vi "Rectangel StraightenLineBetweenRectangles.vi"(1 "Rect1ConnectionOffset":cluster{"x":i32, "y":i32}, 2 "Rect1":T3 {"height" format="%.2f"; "width" format="%.2f"; "y" format="%.2f"; "x" format="%.2f"}, 3 "Rect2ConnectionOffset":cluster{"x":i32, "y":i32}, 4 "Rect2":T3 {"height" format="%.2f"; "width" format="%.2f"; "y" format="%.2f"; "x" format="%.2f"}, 5 "error in (no error)":errorcluster, 6 "Rect1LineDirection":T2, 7 "Rect2LineDirection":T2, 9 "path":T1[](array[typedef]) {"y" format="%.2f"; "x" format="%.2f"}) -> (14 "AdjustmentOK":bool, 15 "Rect1ConnectionOffset":cluster{"x":i32, "y":i32}, 16 "Rect2ConnectionOffset":cluster{"x":i32, "y":i32}, 19 "error out":errorcluster)   [LabVIEW 2014]
doc: "contains"
uses:
  <resource>/Framework/Providers/Open_GDS/UML/General/Rectangle/Rectangle Rectangle2D.ctl
  <resource>/Framework/Providers/Open_GDS/UML/Direction_class/DirectionTypes.ctl
  <resource>/Framework/Providers/Open_GDS/UML/General/Point/Point Point2D.ctl
  <resource>/Framework/Providers/Open_GDS/UML/Direction_class/Direction.lvclass
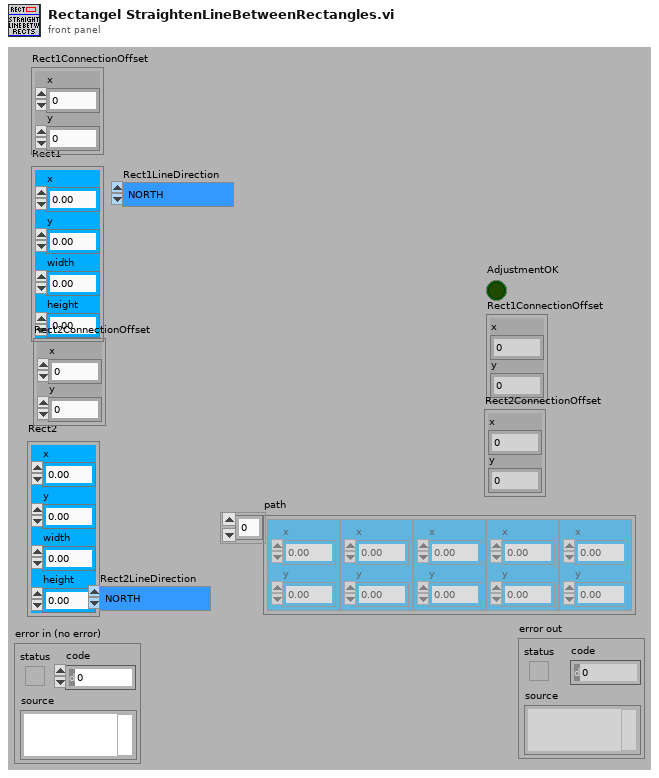
[diagram p1: front panel]
types:
  T1 = typedef "Point Point2D.ctl" = cluster{"x":dbl, "y":dbl}
  T2 = typedef "Direction.lvclass/DirectionTypes.ctl" = enum16{"NORTH", "SOUTH", "EAST", "WEST"}
  T3 = typedef "Rectangle Rectangle2D.ctl" = cluster{"x":dbl, "y":dbl, "width":dbl, "height":dbl}
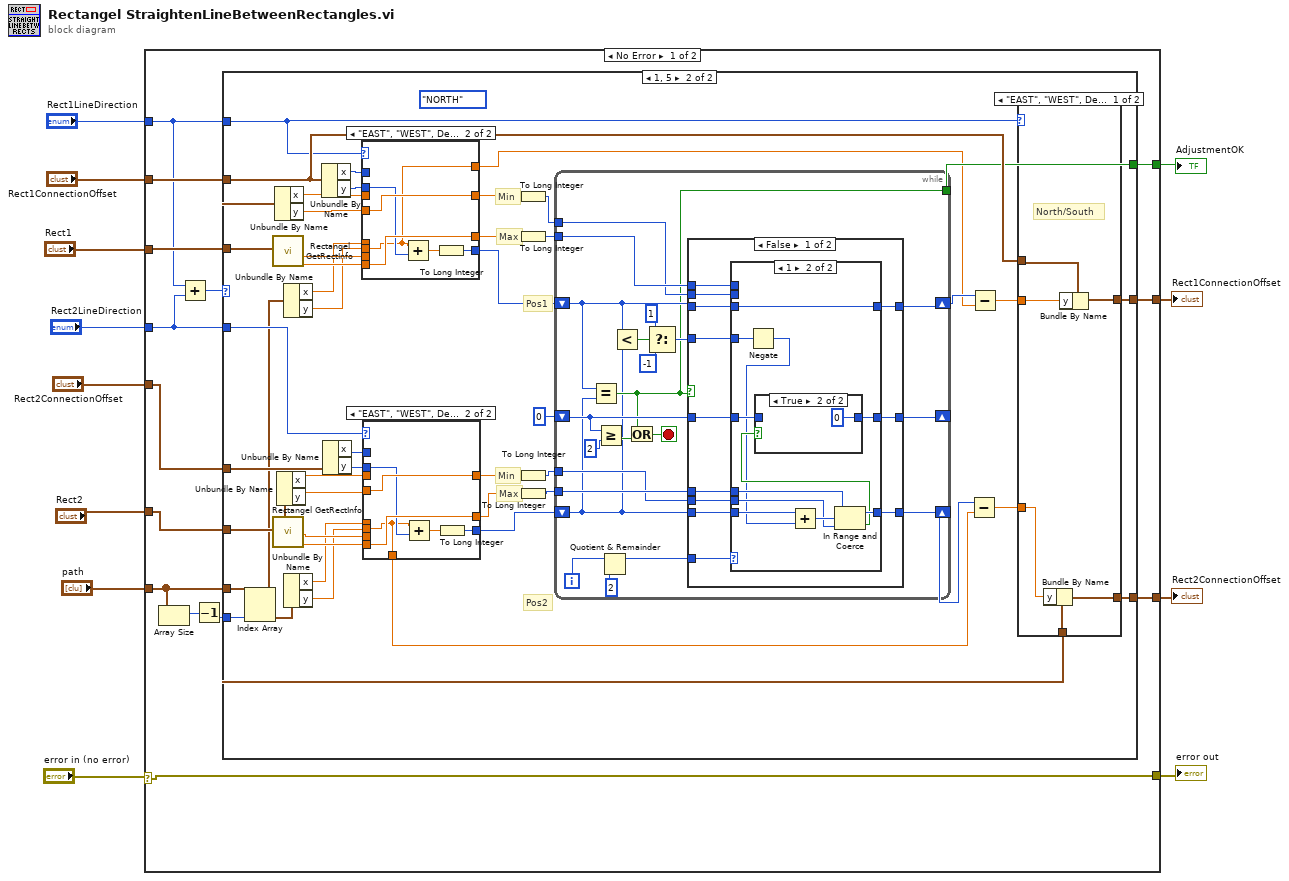
[diagram p0: block diagram]
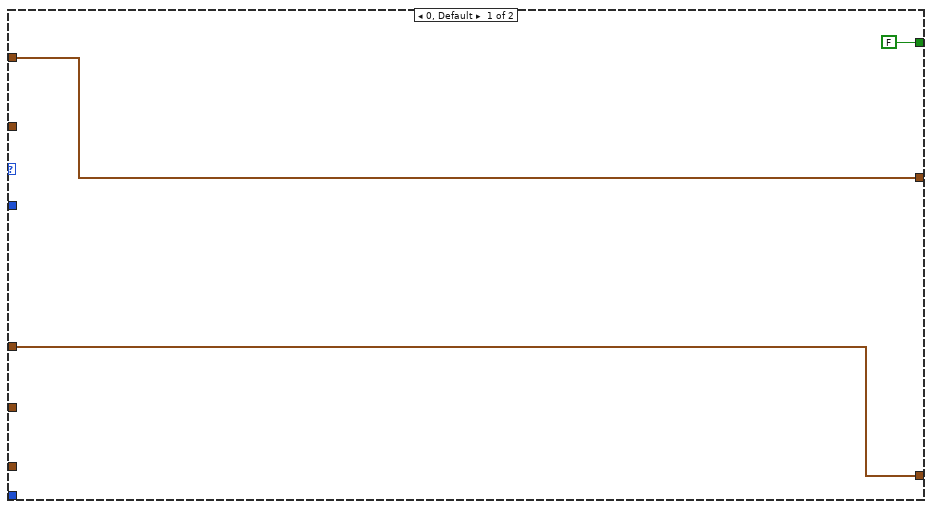
[diagram p2: hidden frame]
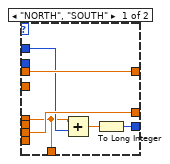
[diagram p3: hidden frame]
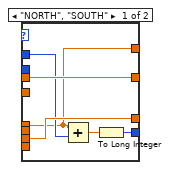
[diagram p4: hidden frame]
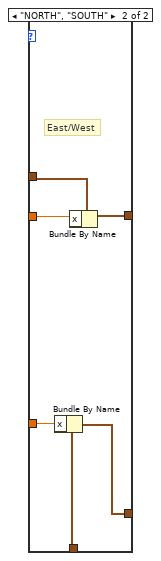
[diagram p5: hidden frame]
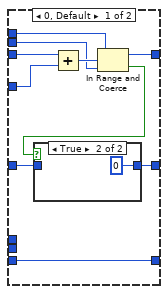
[diagram p6: hidden frame]
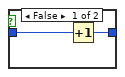
[diagram p7: hidden frame]
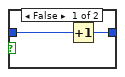
[diagram p8: hidden frame]
diagram:
  n1 = case shown="No Error" "error in (no error)" {
    selector: "error in (no error)" -> [w26 w175]
    tunnel: [w26 w175] -> w12
    tunnel: "Rect1" -> [w22 _]
    tunnel: "Rect1ConnectionOffset" -> [w23 _]
    tunnel: [w25 _] -> w8
    tunnel: "Rect2ConnectionOffset" -> [w19 _]
    tunnel: [w24 _] -> w6
    tunnel: "Rect1LineDirection" -> [w18 _]
    tunnel: [w21 _] -> w4
    tunnel: "Rect2" -> [w20 _]
    tunnel: "Rect2LineDirection" -> [w17 _]
    tunnel: "path" -> [w15 _]
    frame No Error {
      n2 = Array Size(array=w15) -> (size(s)=w14:i32)
      n3 = Add(x=w18, y=w17) -> (x+y=w16:u16)
      n4 = Decrement(x=w14) -> (x-1=w13:i32)
      n5 = case shown="1, 5" w16 {
        tunnel: [w28 w75] -> w25
        tunnel: [w27 w73] -> w24
        tunnel: w23 -> [w28 w72]
        tunnel: w22 -> [_ w70]
        tunnel: [FALSE w64] -> w21
        tunnel: w20 -> [_ w62]
        tunnel: w19 -> [w27 w61]
        tunnel: w18 -> [_ w44]
        tunnel: w17 -> [_ w51]
        tunnel: w15 -> [_ w37]
        tunnel: w13 -> [_ w36]
        frame 0, Default {
        }
        frame 1, 5 {
          (unwired) DirectionTypes."NORTH" ("Rect1LineDirection")
          # "Max"
          # "Min"
          # "Max"
          # "Min"
          # "Pos2"
          # "Pos1"
          n6 = Index Array(array=w37, index #2=w36) -> (element #1=w35:T1, element #2=w32:T1)  [unwired: 1 in]
          n7 = call <resource>:"Rectangel GetRectInfo.vi"("bounds"=w70) -> ("maxX"=w68:dbl, "maxY"=w58:dbl)  [unwired: 1 in, 16 out]
          n8 = call <resource>:"Rectangel GetRectInfo.vi"("bounds"=w62) -> ("maxX"=w53:dbl, "maxY"=w52:dbl)  [unwired: 1 in, 16 out]
          n9 = Unbundle By Name(w70) -> ("x"=w69:dbl, "y"=w59:dbl)
          n10 = Unbundle By Name(w62) -> ("x"=w55:dbl, "y"=w54:dbl)
          n11 = Unbundle By Name(w35) -> ("x"=w33:dbl, "y"=w34:dbl)
          n12 = Unbundle By Name(w32) -> ("x"=w31:dbl, "y"=w30:dbl)
          n13 = Unbundle By Name(w72) -> ("x"=w71:i32, "y"=w60:i32)
          n14 = Unbundle By Name(w61) -> ("x"=w57:i32, "y"=w56:i32)
          n15 = case shown="\"EAST\", \"WEST\", Default" w44 {
            tunnel: w71 -> [w89 _]
            tunnel: w33 -> [w88 _]
            tunnel: [w92 w98] -> w39
            tunnel: w69 -> [w91 _]
            tunnel: w68 -> [w90 _]
            tunnel: [w91 w97] -> w67
            tunnel: [w90 w96] -> w66
            tunnel: w60 -> [_ w95]
            tunnel: w59 -> [_ w97]
            tunnel: w34 -> [_ w94]
            tunnel: w58 -> [_ w96]
            tunnel: [w88 w94] -> w40
            frame "NORTH", "SOUTH" {
              n16 = Add(x=w88, y=w89) -> (x+y=w93:dbl)
              n17 = To Long Integer(number=w93) -> (32bit integer=w92:i32)
            }
            frame "EAST", "WEST", Default {
              n18 = Add(x=w94, y=w95) -> (x+y=w99:dbl)
              n19 = To Long Integer(number=w99) -> (32bit integer=w98:i32)
            }
          }
          n20 = case shown="\"EAST\", \"WEST\", Default" w51 {
            tunnel: w57 -> [w77 _]
            tunnel: w31 -> [w76 _]
            tunnel: [w80 w86] -> w41
            tunnel: w55 -> [w79 _]
            tunnel: w53 -> [w78 _]
            tunnel: [w79 w85] -> w49
            tunnel: [w78 w84] -> w48
            tunnel: w56 -> [_ w83]
            tunnel: w54 -> [_ w85]
            tunnel: w30 -> [_ w82]
            tunnel: w52 -> [_ w84]
            tunnel: [w76 w82] -> w38
            frame "NORTH", "SOUTH" {
              n21 = Add(x=w76, y=w77) -> (x+y=w81:dbl)
              n22 = To Long Integer(number=w81) -> (32bit integer=w80:i32)
            }
            frame "EAST", "WEST", Default {
              n23 = Add(x=w82, y=w83) -> (x+y=w87:dbl)
              n24 = To Long Integer(number=w87) -> (32bit integer=w86:i32)
            }
          }
          n25 = To Long Integer(number=w67) -> (32bit integer=w50:i32)
          n26 = To Long Integer(number=w66) -> (32bit integer=w65:i32)
          n27 = To Long Integer(number=w49) -> (32bit integer=w46:i32)
          n28 = To Long Integer(number=w48) -> (32bit integer=w47:i32)
          n29 = while {
            shift-right: [w122] -> w43
            shift-left: w39 -> [w129]
            shift-right: [w121] -> w42
            shift-left: w41 -> [w112]
            tunnel: w50 -> [w123]
            tunnel: w65 -> [w124]
            shift-right: [w120] -> _
            shift-left: 0 -> [w119]
            tunnel: [w115] -> w64
            tunnel: w47 -> [w114]
            tunnel: w46 -> [w113]
            i -> [w132]
            stop <- w116 stop-if-true
            n30 = Equal?(x=w129, y=w112) -> (x = y?=w115:bool)
            n31 = Greater Or Equal?(x=w119, y=2) -> (x >= y?=w117:bool)
            n32 = Quotient & Remainder(x=w132, y=2) -> (x-y*floor(x/y)=w130:i32)  [unwired: 1 out]
            n33 = Less?(x=w129, y=w112) -> (x < y?=w128:bool)
            n34 = Or(x=w115, y=w117) -> (x .or. y?=w116:bool)
            n35 = Select(t=1, s=w128, f=-1) -> (s? t:f=w125:i32)
            n36 = case shown="False" w115 {
              tunnel: w130 -> [w144 _]
              tunnel: w129 -> [w143 w172]
              tunnel: w125 -> [w142 _]
              tunnel: w124 -> [w141 _]
              tunnel: w123 -> [w140 _]
              tunnel: [w139 w172] -> w122
              tunnel: [w138 w174] -> w121
              tunnel: [w137 w173] -> w120
              tunnel: w119 -> [w136 w173]
              tunnel: w114 -> [w135 _]
              tunnel: w113 -> [w134 _]
              tunnel: w112 -> [w133 w174]
              frame False {
                n37 = case shown="1" w144 {
                  tunnel: w143 -> [w154 w158]
                  tunnel: w142 -> [w153 w160]
                  tunnel: w141 -> [w151 _]
                  tunnel: w140 -> [w150 _]
                  tunnel: [w149 w158] -> w139
                  tunnel: [w148 w167] -> w138
                  tunnel: [w145 w165] -> w137
                  tunnel: w136 -> [w146 w164]
                  tunnel: w135 -> [_ w163]
                  tunnel: w134 -> [_ w162]
                  tunnel: w133 -> [w148 w161]
                  frame 0, Default {
                    n38 = Add(x=w154, y=w153) -> (x+y=w152:i32)
                    n39 = In Range and Coerce(upper limit=w151, x=w152, lower limit=w150) -> (coerced(x)=w149:i32, In Range?=w147:bool)
                    n40 = case shown="True" w147 {
                      tunnel: [w156 0] -> w145
                      tunnel: w146 -> [w155 _]
                      frame False {
                        n41 = Increment(x=w155) -> (x+1=w156:i32)
                      }
                      frame True {
                      }
                    }
                  }
                  frame 1 {
                    n42 = Negate(x=w160) -> (-x=w159:i32)
                    n43 = Add(x=w161, y=w159) -> (x+y=w168:i32)
                    n44 = In Range and Coerce(upper limit=w163, x=w168, lower limit=w162) -> (coerced(x)=w167:i32, In Range?=w166:bool)
                    n45 = case shown="True" w166 {
                      tunnel: [w170 0] -> w165
                      tunnel: w164 -> [w169 _]
                      frame False {
                        n46 = Increment(x=w169) -> (x+1=w170:i32)
                      }
                      frame True {
                      }
                    }
                  }
                }
              }
              frame True {
              }
            }
          }
          n47 = Subtract(x=w42, y=w38) -> (x-y=w74:dbl)
          n48 = Subtract(x=w43, y=w40) -> (x-y=w45:dbl)
          n49 = case shown="\"EAST\", \"WEST\", Default" w44 {
            tunnel: w72 -> [w105 w111]
            tunnel: [w104 w110] -> w75
            tunnel: w74 -> [w103 w109]
            tunnel: w61 -> [w102 w108]
            tunnel: [w101 w107] -> w73
            tunnel: w45 -> [w100 w106]
            frame "EAST", "WEST", Default {
              # "North/South"
              n50 = Bundle By Name(cluster=w102, "y"=w103) -> (w101:cluster{"x":i32, "y":i32})
              n51 = Bundle By Name(cluster=w105, "y"=w100) -> (w104:cluster{"x":i32, "y":i32})
            }
            frame "NORTH", "SOUTH" {
              # "East/West"
              n52 = Bundle By Name(cluster=w108, "x"=w109) -> (w107:cluster{"x":i32, "y":i32})
              n53 = Bundle By Name(cluster=w111, "x"=w106) -> (w110:cluster{"x":i32, "y":i32})
            }
          }
        }
      }
    }
    frame Error {
    }
  }
  "error out" <- w12
  "Rect2ConnectionOffset" <- w6
  "Rect1ConnectionOffset" <- w8
  "AdjustmentOK" <- w4
